vi "GUI.Settings.vi"(8 "error in":errorcluster) -> (0 "error out":errorcluster, 3 "Setting Options":T1)   [LabVIEW 2022 SP3]
panel:
  # "Settings"
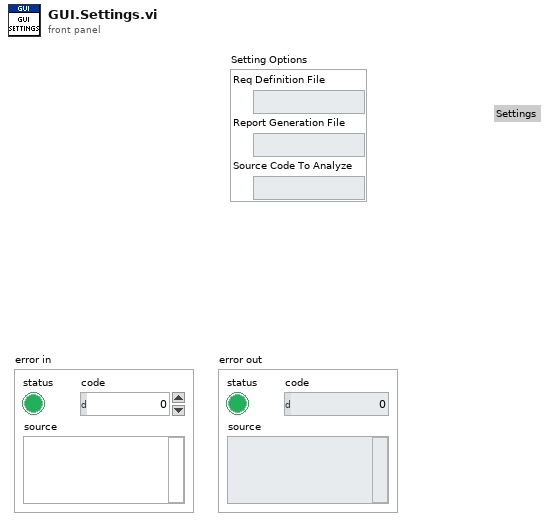
[diagram p1: front panel]
types:
  T1 = cluster{"Req Definition File":path, "Report Generation File":path, "Source Code To Analyze":path}
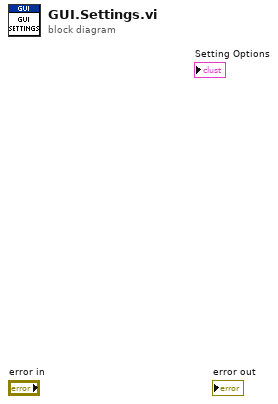
[diagram p0: block diagram]
diagram:
